vi "CreateFileVersionTxt.vi"   [LabVIEW 2013, in "main.lvlib"]
uses:
  main.lvlib
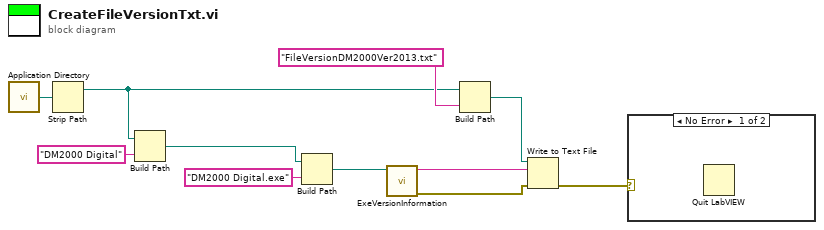
[diagram p0: block diagram]
diagram:
  n1 = call <vilib>:"Application Directory.vi"() -> ("Application Directory"=w4:path)
  n2 = Strip Path(path=w4) -> (stripped path=w1:path)  [unwired: 1 out]
  n3 = Build Path(base path=w1, name or relative path="DM2000 Digital") -> (appended path=w2:path)
  n4 = Build Path(base path=w2, name or relative path="DM2000 Digital.exe") -> (appended path=w6:path)
  n5 = call "ExeVersionInformation.vi"("path"=w6) -> ("error out"=w11:errorcluster, "FileVersion"=w8:string)  [unwired: 9 in]
  n6 = Build Path(base path=w1, name or relative path="FileVersionDM2000Ver2013.txt") -> (appended path=w10:path)
  n7 = Write to Text File(file (use dialog)=w10, text=w8, error in=w11) -> (error out=w5:errorcluster)  [unwired: 1 in, 2 out]
  n8 = case shown="No Error" w5 {
    frame No Error {
      n9 = Quit LabVIEW() -> ()  [unwired: 1 in]
    }
    frame Error {
    }
  }
